vi "T90 Anpassung LP.vi"(0 "DO 0-31":T1, 11 "error in (no error)":errorcluster caption="Fehler (Eingang, kein Fehler)") -> (4 "DO 0-31":T1, 15 "error out":errorcluster caption="Fehler (Ausgang)")   [LabVIEW 2020, in "Allgemein.lvlib"]
uses:
  Allgemein.lvlib
  Aktion FGV T90.ctl
  Verwaltung/Digital Ausgaenge 0-31.ctl
  Verwaltung/Verwaltung - cRIO.lvlib
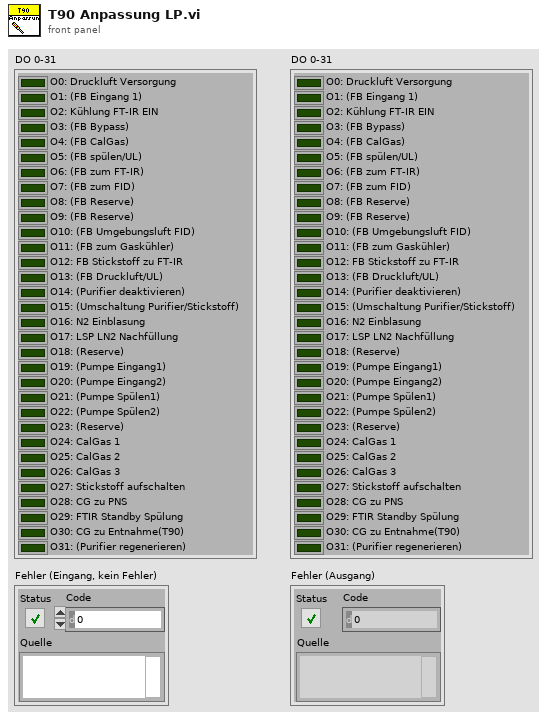
[diagram p1: front panel]
types:
  T1 = typedef "Verwaltung - cRIO.lvlib/Digital Ausgaenge 0-31.ctl" = cluster{"O0: Druckluft Versorgung":bool, "O1: (FB Eingang 1)":bool, "O2: Kühlung FT-IR EIN":bool, "O3: (FB Bypass)":bool, "O4: (FB CalGas)":bool, "O5: (FB spülen/UL)":bool, "O6: (FB zum FT-IR)":bool, "O7: (FB zum FID)":bool, "O8: (FB Reserve)":bool, "O9: (FB Reserve)":bool, "O10: (FB Umgebungsluft FID)":bool, "O11: (FB zum Gaskühler)":bool, "O12: FB Stickstoff zu FT-IR":bool, "O13: (FB Druckluft/UL)":bool, "O14: (Purifier deaktivieren)":bool, "O15: (Umschaltung Purifier/Stickstoff)":bool, "O16: N2 Einblasung":bool, "O17: LSP LN2 Nachfüllung":bool, "O18: (Reserve)":bool, "O19: (Pumpe Eingang1)":bool, "O20: (Pumpe Eingang2)":bool, "O21: (Pumpe Spülen1)":bool, "O22: (Pumpe Spülen2)":bool, "O23: (Reserve)":bool, "O24: CalGas 1":bool, "O25: CalGas 2":bool, "O26: CalGas 3":bool, "O27: Stickstoff aufschalten":bool, "O28: CG zu PNS":bool, "O29: FTIR Standby Spülung":bool, "O30: CG zu Entnahme(T90)":bool, "O31: (Purifier regenerieren)":bool}
  T2 = typedef "Allgemein.lvlib/Aktion FGV T90.ctl" = enum16{"lesen", "schreiben"}
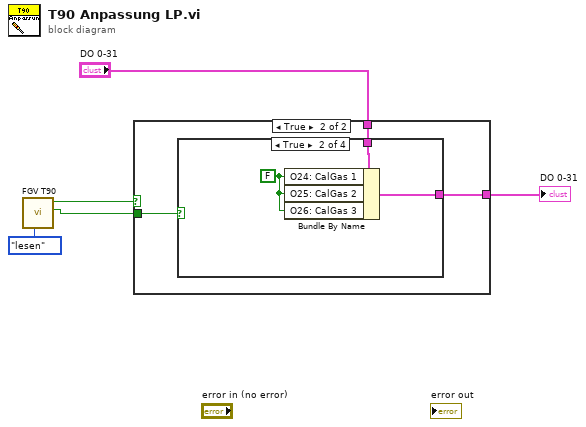
[diagram p0: block diagram]
diagram:
  n1 = call "FGV T90.vi"("Aktion"=Aktion_FGV_T90."lesen") -> ("N2 Spülen aktiv"=w1:bool, "T90 aktiv"=w2:bool)  [unwired: 7 in, 2 out]
  n2 = case shown="True" w2 {
    tunnel: "DO 0-31" -> [w6 w9]
    tunnel: [w6 w8] -> w4
    tunnel: w1 -> [_ w7]
    frame False {
    }
    frame True {
      n3 = case shown="\"Warten\"" w7 {
        tunnel: w9 -> [w10 w13 w14 w15]
        tunnel: [w10 w12 w14 w15] -> w8
        frame True {
        }
        frame True {
          w11 = FALSE ("O24: CalGas 1")
          n4 = Bundle By Name(cluster=w13, "O24: CalGas 1"=w11, "O25: CalGas 2"=w11, "O26: CalGas 3"=w11) -> (w12:T1)
        }
        frame False {
        }
        frame True {
        }
      }
    }
  }
  "DO 0-31" <- w4
